vi "test-Diff-Drive-Accel-Limiter-Test1.vi"(8 "error in (no error)":errorcluster) -> (0 "error out":errorcluster, 3 "All tests passed":bool)   [LabVIEW 2019]
uses:
  <vilib>/Analysis/baseanly.llb/Real A x B.vi
  <vilib>/Rock Robotics/WPI/ThirdParty/JAS_Junk/TrajLib/MatBuilder_Create.vi
  <vilib>/Rock Robotics/WPI/ThirdParty/JAS_Junk/TrajLib/LinearSystem_New.vi
  <vilib>/Rock Robotics/WPI/ThirdParty/JAS_Junk/TrajLib/MatrixHelper_Zero.vi
  <vilib>/Rock Robotics/WPI/ThirdParty/JAS_Junk/TrajLib/Discretization_DiscretizeAB.vi
  <vilib>/Rock Robotics/WPI/ThirdParty/JAS_Junk/TrajLib/MatrixHelper_CoerceSize.vi
  <vilib>/Rock Robotics/WPI/ThirdParty/JAS_Junk/TrajLib/Matrix_Exp.vi
  <vilib>/Rock Robotics/WPI/ThirdParty/JAS_Junk/TrajLib/Matrix_AssignBlock.vi
  <vilib>/Rock Robotics/WPI/ThirdParty/JAS_Junk/TrajLib/Matrix_ExtractFrom.vi
  <vilib>/Analysis/7linalg.llb/Matrix Exp.vi
  <vilib>/Analysis/7linalg.llb/Real Matrix Exp.vi
  <vilib>/Analysis/Matrix/Numeric/Add/Add - RM,RM.vi
  <vilib>/Analysis/Matrix/Numeric/Multiply/Multiply.vi
  <vilib>/Analysis/Matrix/Numeric/Multiply/Multiply - RM,R.vi
  <vilib>/Rock Robotics/WPI/ThirdParty/JAS_Junk/TrajLib/Trajectory_Library.lvlib
  <vilib>/Analysis/NI_AALBase.lvlib
  <vilib>/Analysis/Matrix/NI_Matrix.lvlib
panel:
  out "max value 6":dbl
  out "max value 5":dbl
  out "max value 4":dbl
  out "max value 3":dbl
  out "max value 2":dbl
  out "max value":dbl
  out "Test 1":bool
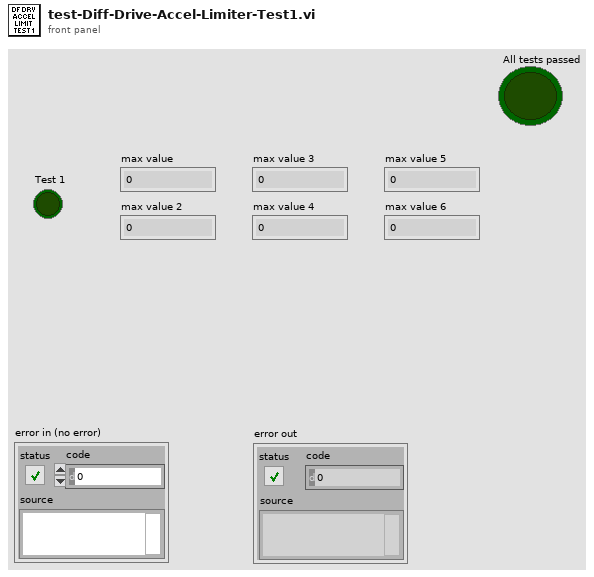
[diagram p1: front panel]
types:
  T1 = typedef "NI_Matrix.lvlib/RealMatrix.ctl" = dbl[][]
  T2 = typedef "Trajectory_Library.lvlib/LINEAR_SYSTEM.ctl" = cluster{"m_A":T1, "m_B":T1, "m_C":T1, "m_D":T1, "States":i32, "Inputs":i32, "Outputs":i32}
  T3 = typedef "Trajectory_Library.lvlib/DIFF_DRIVE_ACCEL_LIMIT.ctl" = cluster{"m_system":T2, "m_trackwidth":dbl, "m_maxLinearAccel":dbl, "m_maxAngularAccel":dbl}
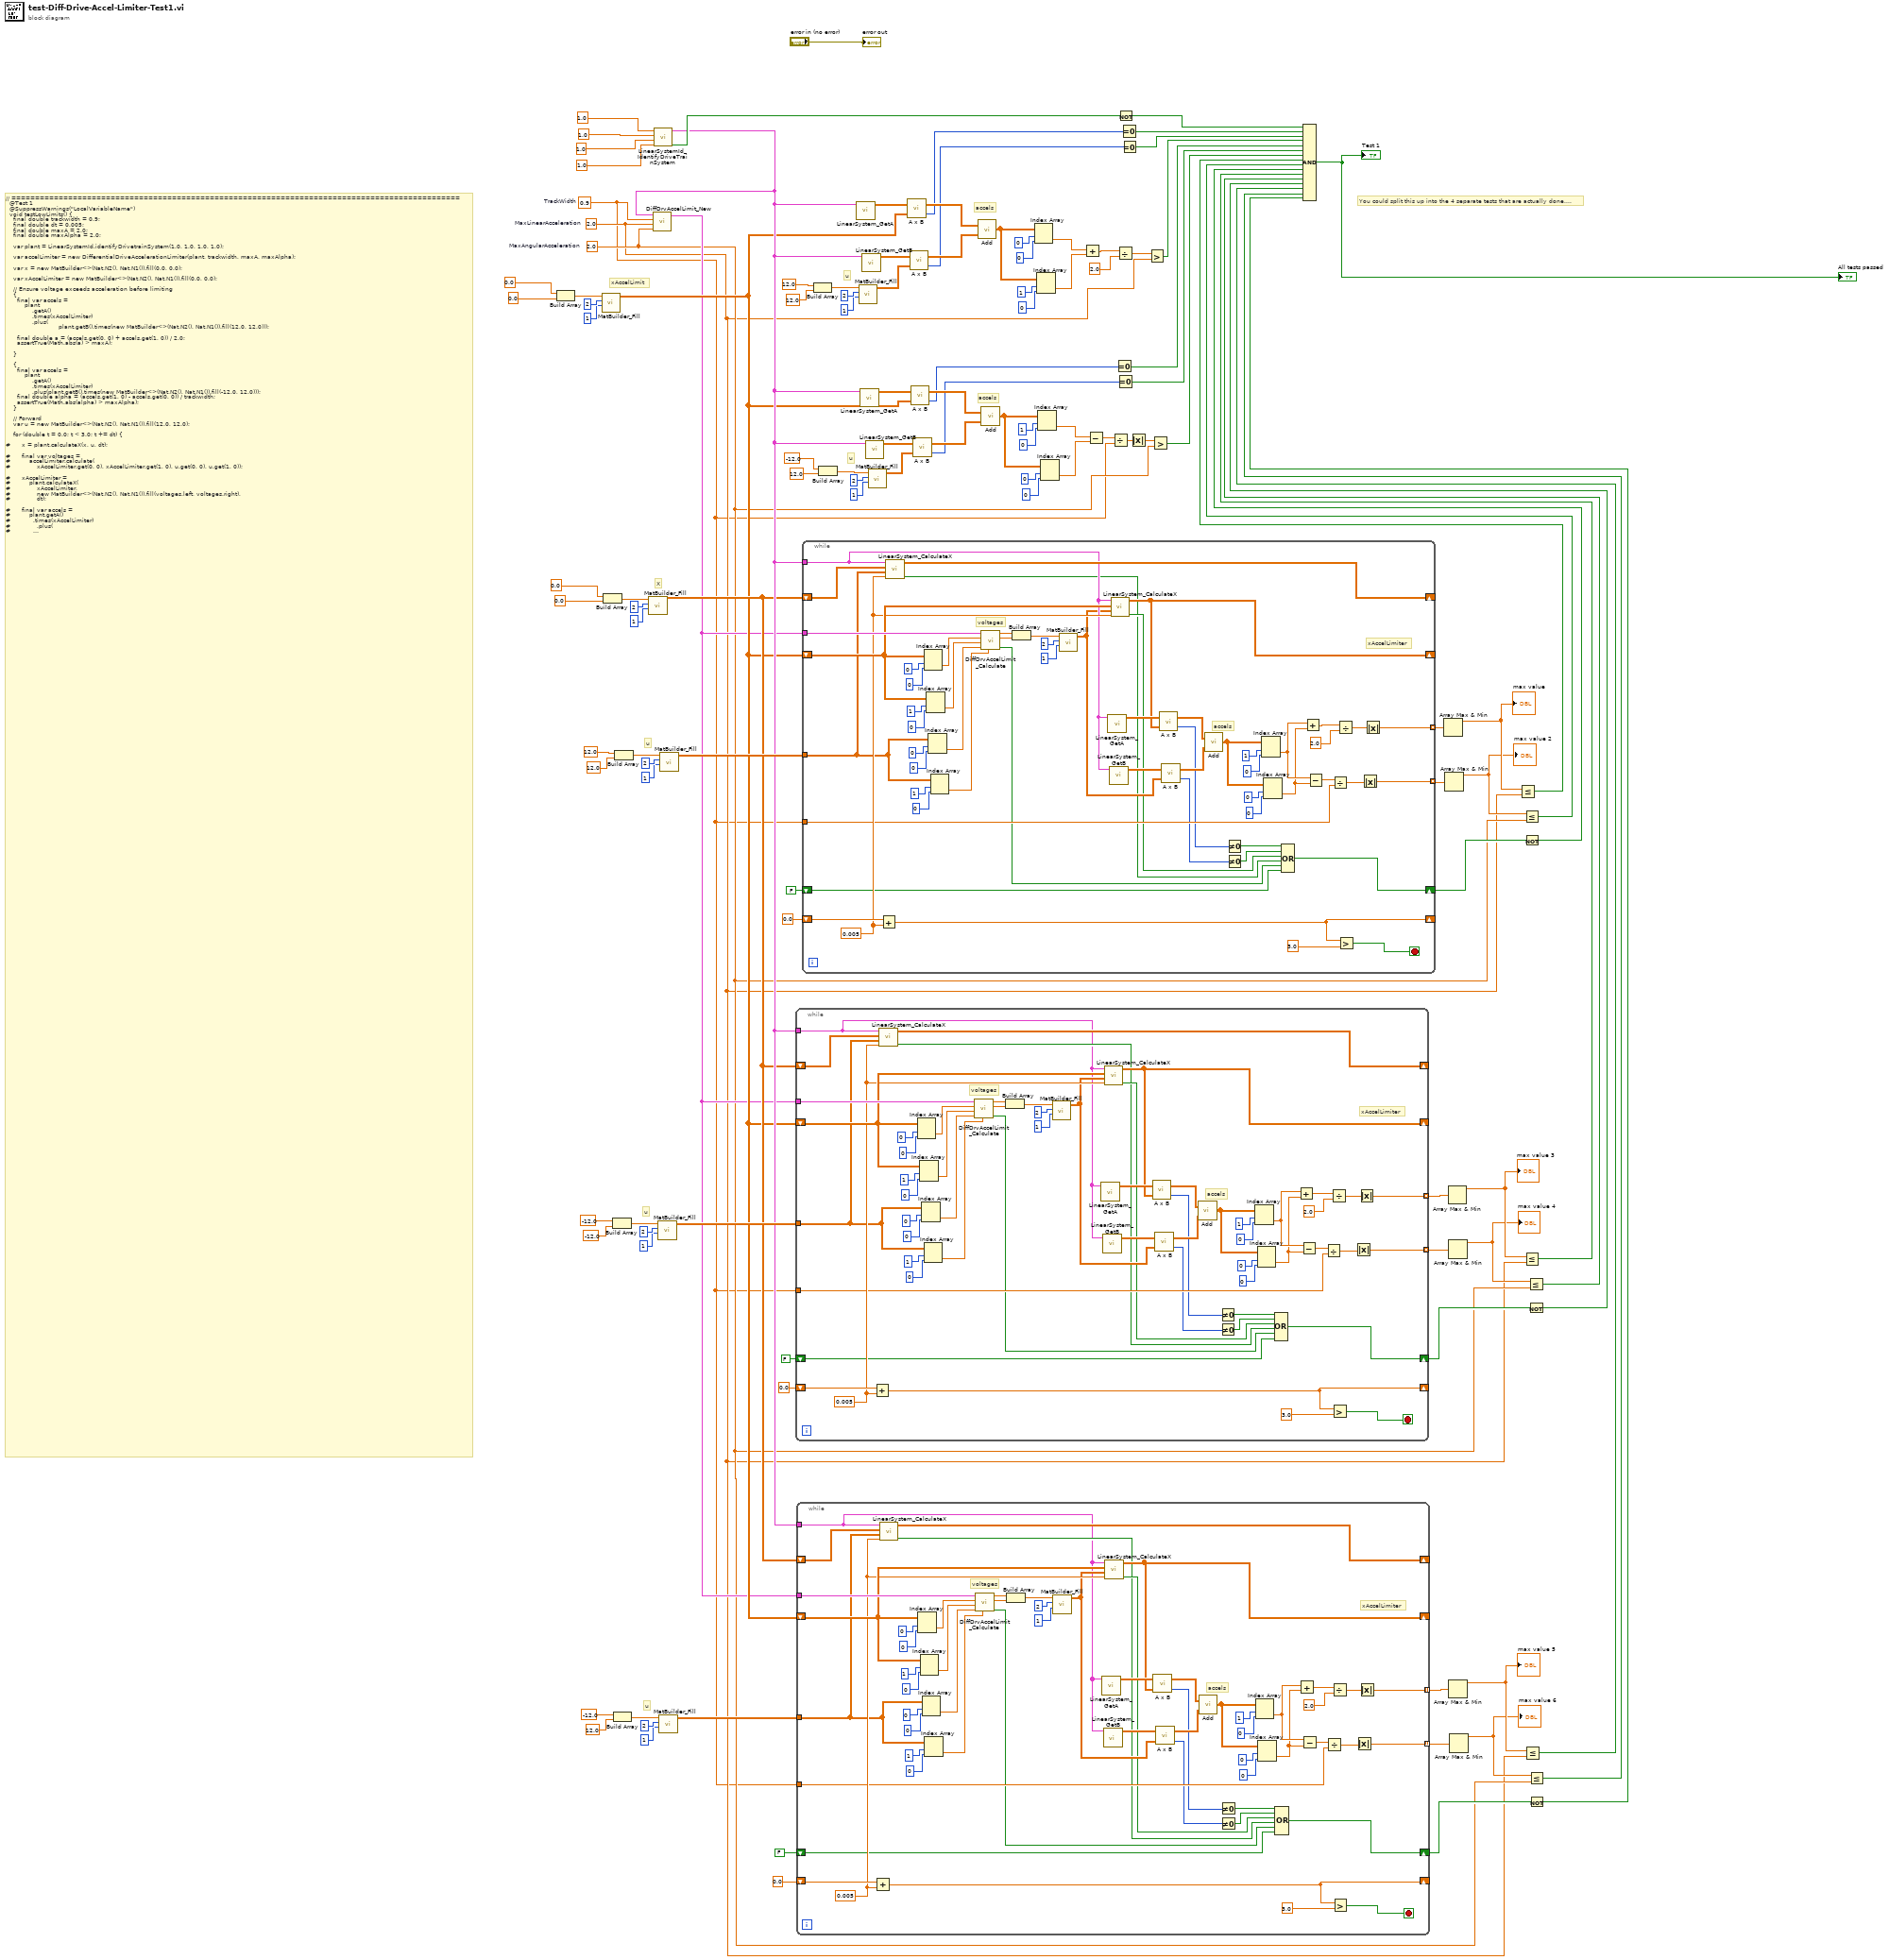
[diagram p0: block diagram]
diagram:
  w5 = 0.9  # TrackWidth
  w6 = 2.0  # MaxLinearAcceleration
  w7 = 2.0  # MaxAngularAcceleration
  # "You could split this up into the 4 separate tests that are actually done...."
  # "u"
  # "u"
  # "u"
  # "u"
  # "u"
  # "accels"
  # "accels"
  # "xAccelLimit"
  # "X"
  # "// ===============================================================================================\n  @Test 1\n  @SuppressWarnings(\"LocalVariableName\")\n  void testLowLimits() {\n    final double trackwidth = 0.9;\n    final double dt = 0.005;\n    final double maxA = 2.0;\n    final double maxAlpha = 2.0;\n\n    var plant = LinearSystemId.identifyDrivetrainSystem(1.0, 1.0, 1.0, 1.0);\n\n    var accelLimiter = new DifferentialDriveAccelerationLimiter(plant, trackwidth, maxA, maxAlpha);\n\n    var x = new MatBuilder<>(Nat.N2(), Nat.N1()).fill(0.0, 0.0);\n\n    var xAccelLimiter = new MatBuilder<>(Nat.N2(), Nat.N1()).fill(0.0, 0.0);\n\n    // Ensure voltage exceeds acceleration before limiting\n    {\n      final var accels =\n          plant\n              .getA()\n              .times(xAccelLimiter)\n              .plus(\n                            plant.getB().times(new MatBuilder<>(Nat.N2(), Nat.N1()).fill(12.0, 12.0)));\n\n      final double a = (accels.get(0, 0) + accels.get(1, 0)) / 2.0;\n      assertTrue(Math.abs(a) > maxA);\n\n    }\n\n    {\n      final var accels =\n          plant\n              .getA()\n              .times(xAccelLimiter)\n              .plus(plant.getB().times(new MatBuilder<>(Nat.N2(), Nat.N1()).fill(-12.0, 12.0)));\n      final double alpha = (accels.get(1, 0) - accels.get(0, 0)) / trackwidth;\n      assertTrue(Math.abs(alpha) > maxAlpha);\n    }\n\n    // Forward\n    var u = new MatBuilder<>(Nat.N2(), Nat.N1()).fill(12.0, 12.0);\n\n    for (double t = 0.0; t < 3.0; t += dt) {\n\n#      x = plant.calculateX(x, u, dt);\n\n#      final var voltages =\n#          accelLimiter.calculate(\n#              xAccelLimiter.get(0, 0), xAccelLimiter.get(1, 0), u.get(0, 0), u.get(1, 0));\n\n#      xAccelLimiter =\n#          plant.calculateX(\n#              xAccelLimiter,\n#              new MatBuilder<>(Nat.N2(), Nat.N1()).fill(voltages.left, voltages.right),\n#              dt);\n\n#      final var accels =\n#          plant.getA()\n#            .times(xAccelLimiter)\n#              .plus(\n#                  plant.getB()\n#                      .times(\n#                          new MatBuilder<>(Nat.N2(), Nat.N1())\n#                              .fill(voltages.left, voltages.right)));\n\n#      final double a = (accels.get(0, 0) + accels.get(1, 0)) / 2.0;\n\n#      final double alpha = (accels.get(1, 0) - accels.get(0, 0)) / trackwidth;\n\n#      assertTrue(Math.abs(a) <= maxA);\n#      assertTrue(Math.abs(alpha) <= maxAlpha);\n\n#    }\n\n    // Backward\n    u = new MatBuilder<>(Nat.N2(), Nat.N1()).fill(-12.0, -12.0);\n\n    for (double t = 0.0; t < 3.0; t += dt) {\n      x = plant.calculateX(x, u, dt);\n      final var voltages =\n          accelLimiter.calculate(\n              xAccelLimiter.get(0, 0), xAccelLimiter.get(1, 0), u.get(0, 0), u.get(1, 0));\n      xAccelLimiter =\n          plant.calculateX(\n              xAccelLimiter,\n              new MatBuilder<>(Nat.N2(), Nat.N1()).fill(voltages.left, voltages.right),\n              dt);\n\n      final var accels =\n          plant\n              .getA()\n              .times(xAccelLimiter)\n              .plus(\n                  plant\n                      .getB()\n                      .times(\n                          new MatBuilder<>(Nat.N2(), Nat.N1())\n                              .fill(voltages.left, voltages.right)));\n\n      final double a = (accels.get(0, 0) + accels.get(1, 0)) / 2.0;\n\n      final double alpha = (accels.get(1, 0) - accels.get(0, 0)) / trackwidth;\n\n      assertTrue(Math.abs(a) <= maxA);\n      assertTrue(Math.abs(alpha) <= maxAlpha);\n    }\n\n\n    // Rotate CCW\n    u = new MatBuilder<>(Nat.N2(), Nat.N1()).fill(-12.0, 12.0);\n    for (double t = 0.0; t < 3.0; t += dt) {\n      x = plant.calculateX(x, u, dt);\n      final var voltages =\n          accelLimiter.calculate(\n              xAccelLimiter.get(0, 0), xAccelLimiter.get(1, 0), u.get(0, 0), u.get(1, 0));\n      xAccelLimiter =\n          plant.calculateX(\n              xAccelLimiter,\n              new MatBuilder<>(Nat.N2(), Nat.N1()).fill(voltages.left, voltages.right),\n              dt);\n\n      final var accels =\n          plant\n              .getA()\n              .times(xAccelLimiter)\n              .plus(\n                  plant\n                      .getB()\n                      .times(\n                          new MatBuilder<>(Nat.N2(), Nat.N1())\n                              .fill(voltages.left, voltages.right)));\n      final double a = (accels.get(0, 0) + accels.get(1, 0)) / 2.0;\n      final double alpha = (accels.get(1, 0) - accels.get(0, 0)) / trackwidth;\n      assertTrue(Math.abs(a) <= maxA);\n      assertTrue(Math.abs(alpha) <= maxAlpha);\n    }\n  }"
  n1 = Build Array(0.0 ("element"), 0.0 ("element")) -> (w113:dbl[])
  n2 = call <vilib>:"MatBuilder_Fill.vi"("Columns"=1, "Rows"=2, "Value List"=w113) -> ("output matrix"=w9:T1)  [unwired: 8 in]
  n3 = Build Array(0.0 ("element"), 0.0 ("element")) -> (w118:dbl[])
  n4 = Build Array(-12.0 ("element"), -12.0 ("element")) -> (w38:dbl[])
  n5 = Build Array(-12.0 ("element"), 12.0 ("element")) -> (w22:dbl[])
  n6 = Build Array(12.0 ("element"), 12.0 ("element")) -> (w56:dbl[])
  n7 = call <vilib>:"MatBuilder_Fill.vi"("Columns"=1, "Rows"=2, "Value List"=w118) -> ("output matrix"=w10:T1)  [unwired: 8 in]
  n8 = call <vilib>:"LinearSystemId_IdentifyDriveTrainSystem.vi"("kAAngular"=1.0 ("rbMeters"), "kVAngular"=1.0 ("rMeters"), "kALinear"=1.0 ("MassKg"), "kVLinear"=1.0 ("JKgMetersSquared")) -> ("Size Coerced"=w93:bool, "Linearsystem"=w11:T2)  [unwired: 6 in]
  n9 = call <vilib>:"DiffDrvAccelLimit_New.vi"("MaxAngularAcceleration"=w7, "MaxLinearAcceleration"=w6, "TrackWidth"=w5, "LINEARSYSTEM"=w11) -> ("outDiffDriveAccelLimit"=w8:T3)  [unwired: 7 in]
  n10 = call <vilib>:"MatBuilder_Fill.vi"("Columns"=1, "Rows"=2, "Value List"=w38) -> ("output matrix"=w33:T1)  [unwired: 8 in]
  n11 = call <vilib>:"MatBuilder_Fill.vi"("Columns"=1, "Rows"=2, "Value List"=w22) -> ("output matrix"=w17:T1)  [unwired: 8 in]
  n12 = call <vilib>:"MatBuilder_Fill.vi"("Columns"=1, "Rows"=2, "Value List"=w56) -> ("output matrix"=w50:T1)  [unwired: 8 in]
  n13 = while {
    shift-right: [w178] -> _
    shift-left: 0.0 -> [w181]
    tunnel: w33 -> [w139]
    shift-right: [w171] -> _
    shift-left: w10 -> [w177]
    tunnel: w8 -> [w176]
    shift-right: [w146] -> _
    shift-left: w9 -> [w162]
    tunnel: w5 -> [w138]
    tunnel: [w135] -> w30 mode=indexing
    tunnel: [w134] -> w29 mode=indexing
    shift-right: [w125] -> w28
    shift-left: FALSE -> [w126]
    tunnel: w11 -> [w124]
    stop <- w180 stop-if-true
    w156 = 0.005
    # "voltages"
    # "xAccelLimiter"
    # "accels"
    n14 = Add(x=w181, y=w156) -> (x+y=w178:dbl)
    n15 = call <vilib>:"LinearSystem_CalculateX.vi"("dT_Seconds"=w156, "ClampedU"=w139, "X"=w177, "Linearsystem"=w124) -> ("Error"=w128:bool, "outX"=w171:T1)  [unwired: 6 in]
    n16 = Index Array(array=w162, index (row)=0, index (col)=0) -> (element=w170:dbl)
    n17 = Index Array(array=w162, index (row)=1, index (col)=0) -> (element=w169:dbl)
    n18 = Index Array(array=w139, index (row)=0, index (col)=0) -> (element=w164:dbl)
    n19 = Index Array(array=w139, index (row)=1, index (col)=0) -> (element=w163:dbl)
    n20 = call <vilib>:"DiffDrvAccelLimit_Calculate.vi"("RightVoltage"=w163, "LeftVoltage"=w164, "RightVelocity"=w169, "LeftVelocity"=w170, "inDiffDriveAccelLimit"=w176) -> ("Error"=w127:bool, "NewRightVoltage"=w157:dbl, "NewLeftVoltage"=w158:dbl)  [unwired: 4 in]
    n21 = Build Array(w158, w157) -> (w161:dbl[])
    n22 = call <vilib>:"MatBuilder_Fill.vi"("Columns"=1, "Rows"=2, "Value List"=w161) -> ("output matrix"=w145:T1)  [unwired: 8 in]
    n23 = call <vilib>:"LinearSystem_GetA.vi"("Linearsystem"=w124) -> ("A"=w155:T1)  [unwired: 10 in]
    n24 = call <vilib>:"LinearSystem_GetB.vi"("Linearsystem"=w124) -> ("B"=w154:T1)  [unwired: 10 in]
    n25 = call <vilib>:"LinearSystem_CalculateX.vi"("dT_Seconds"=w156, "ClampedU"=w145, "X"=w162, "Linearsystem"=w124) -> ("Error"=w129:bool, "outX"=w146:T1)  [unwired: 6 in]
    n26 = call-poly <vilib>:"A x B.vi"("B"=w146, "A"=w155) -> ("error"=w132:i32, "A x B"=w153:T1)
    n27 = call-poly <vilib>:"A x B.vi"("B"=w145, "A"=w154) -> ("error"=w131:i32, "A x B"=w152:T1)
    n28 = call-poly <vilib>:"Add.vi"("Real Matrix B"=w152, "Real Matrix A"=w153) -> ("A + B"=w147:T1)
    n29 = Not Equal To 0?(x=w132) -> (x != 0?=w133:bool)
    n30 = Not Equal To 0?(x=w131) -> (x != 0?=w130:bool)
    n31 = Index Array(array=w147, index (row)=1, index (col)=0) -> (element=w141:dbl)
    n32 = Index Array(array=w147, index (row)=0, index (col)=0) -> (element=w140:dbl)
    n33 = Compound Arithmetic op=OR(w133, w130, w129, w128, w127, w126) -> (w125:bool)
    n34 = Add(x=w141, y=w140) -> (x+y=w144:dbl)
    n35 = Subtract(x=w141, y=w140) -> (x-y=w142:dbl)
    n36 = Divide(x=w142, y=w138) -> (x/y=w136:dbl)
    n37 = Divide(x=w144, y=2.0) -> (x/y=w137:dbl)
    n38 = Greater?(x=w178, y=3.0) -> (0:w180:bool)
    n39 = Absolute Value(x=w136) -> (abs(x)=w134:dbl)
    n40 = Absolute Value(x=w137) -> (abs(x)=w135:dbl)
  }
  n41 = while {
    shift-right: [w236] -> _
    shift-left: 0.0 -> [w239]
    tunnel: w17 -> [w197]
    shift-right: [w229] -> _
    shift-left: w10 -> [w235]
    tunnel: w8 -> [w234]
    shift-right: [w204] -> _
    shift-left: w9 -> [w220]
    tunnel: w5 -> [w196]
    tunnel: [w193] -> w14 mode=indexing
    tunnel: [w192] -> w13 mode=indexing
    shift-right: [w183] -> w12
    shift-left: FALSE -> [w184]
    tunnel: w11 -> [w182]
    stop <- w238 stop-if-true
    w214 = 0.005
    # "voltages"
    # "xAccelLimiter"
    # "accels"
    n42 = Add(x=w239, y=w214) -> (x+y=w236:dbl)
    n43 = call <vilib>:"LinearSystem_CalculateX.vi"("dT_Seconds"=w214, "ClampedU"=w197, "X"=w235, "Linearsystem"=w182) -> ("Error"=w186:bool, "outX"=w229:T1)  [unwired: 6 in]
    n44 = Index Array(array=w220, index (row)=0, index (col)=0) -> (element=w228:dbl)
    n45 = Index Array(array=w220, index (row)=1, index (col)=0) -> (element=w227:dbl)
    n46 = Index Array(array=w197, index (row)=0, index (col)=0) -> (element=w222:dbl)
    n47 = Index Array(array=w197, index (row)=1, index (col)=0) -> (element=w221:dbl)
    n48 = call <vilib>:"DiffDrvAccelLimit_Calculate.vi"("RightVoltage"=w221, "LeftVoltage"=w222, "RightVelocity"=w227, "LeftVelocity"=w228, "inDiffDriveAccelLimit"=w234) -> ("Error"=w185:bool, "NewRightVoltage"=w215:dbl, "NewLeftVoltage"=w216:dbl)  [unwired: 4 in]
    n49 = Build Array(w216, w215) -> (w219:dbl[])
    n50 = call <vilib>:"MatBuilder_Fill.vi"("Columns"=1, "Rows"=2, "Value List"=w219) -> ("output matrix"=w203:T1)  [unwired: 8 in]
    n51 = call <vilib>:"LinearSystem_GetA.vi"("Linearsystem"=w182) -> ("A"=w213:T1)  [unwired: 10 in]
    n52 = call <vilib>:"LinearSystem_GetB.vi"("Linearsystem"=w182) -> ("B"=w212:T1)  [unwired: 10 in]
    n53 = call <vilib>:"LinearSystem_CalculateX.vi"("dT_Seconds"=w214, "ClampedU"=w203, "X"=w220, "Linearsystem"=w182) -> ("Error"=w187:bool, "outX"=w204:T1)  [unwired: 6 in]
    n54 = call-poly <vilib>:"A x B.vi"("B"=w204, "A"=w213) -> ("error"=w190:i32, "A x B"=w211:T1)
    n55 = call-poly <vilib>:"A x B.vi"("B"=w203, "A"=w212) -> ("error"=w189:i32, "A x B"=w210:T1)
    n56 = call-poly <vilib>:"Add.vi"("Real Matrix B"=w210, "Real Matrix A"=w211) -> ("A + B"=w205:T1)
    n57 = Not Equal To 0?(x=w190) -> (x != 0?=w191:bool)
    n58 = Not Equal To 0?(x=w189) -> (x != 0?=w188:bool)
    n59 = Index Array(array=w205, index (row)=1, index (col)=0) -> (element=w199:dbl)
    n60 = Index Array(array=w205, index (row)=0, index (col)=0) -> (element=w198:dbl)
    n61 = Compound Arithmetic op=OR(w191, w188, w187, w186, w185, w184) -> (w183:bool)
    n62 = Add(x=w199, y=w198) -> (x+y=w202:dbl)
    n63 = Subtract(x=w199, y=w198) -> (x-y=w200:dbl)
    n64 = Divide(x=w200, y=w196) -> (x/y=w194:dbl)
    n65 = Divide(x=w202, y=2.0) -> (x/y=w195:dbl)
    n66 = Greater?(x=w236, y=3.0) -> (0:w238:bool)
    n67 = Absolute Value(x=w194) -> (abs(x)=w192:dbl)
    n68 = Absolute Value(x=w195) -> (abs(x)=w193:dbl)
  }
  n69 = while {
    shift-right: [w294] -> _
    shift-left: 0.0 -> [w297]
    tunnel: w11 -> [w262]
    tunnel: w50 -> [w254]
    shift-right: [w287] -> _
    shift-left: w10 -> [w293]
    tunnel: w8 -> [w292]
    shift-right: [w261] -> _
    shift-left: w9 -> [w278]
    tunnel: w5 -> [w253]
    tunnel: [w250] -> w49 mode=indexing
    tunnel: [w249] -> w48 mode=indexing
    shift-right: [w240] -> w44
    shift-left: FALSE -> [w241]
    stop <- w296 stop-if-true
    w272 = 0.005
    # "voltages"
    # "xAccelLimiter"
    # "accels"
    n70 = Add(x=w297, y=w272) -> (x+y=w294:dbl)
    n71 = call <vilib>:"LinearSystem_CalculateX.vi"("dT_Seconds"=w272, "ClampedU"=w254, "X"=w293, "Linearsystem"=w262) -> ("Error"=w243:bool, "outX"=w287:T1)  [unwired: 6 in]
    n72 = Index Array(array=w278, index (row)=0, index (col)=0) -> (element=w286:dbl)
    n73 = Index Array(array=w278, index (row)=1, index (col)=0) -> (element=w285:dbl)
    n74 = Index Array(array=w254, index (row)=0, index (col)=0) -> (element=w280:dbl)
    n75 = Index Array(array=w254, index (row)=1, index (col)=0) -> (element=w279:dbl)
    n76 = call <vilib>:"DiffDrvAccelLimit_Calculate.vi"("RightVoltage"=w279, "LeftVoltage"=w280, "RightVelocity"=w285, "LeftVelocity"=w286, "inDiffDriveAccelLimit"=w292) -> ("Error"=w242:bool, "NewRightVoltage"=w273:dbl, "NewLeftVoltage"=w274:dbl)  [unwired: 4 in]
    n77 = Build Array(w274, w273) -> (w277:dbl[])
    n78 = call <vilib>:"MatBuilder_Fill.vi"("Columns"=1, "Rows"=2, "Value List"=w277) -> ("output matrix"=w260:T1)  [unwired: 8 in]
    n79 = call <vilib>:"LinearSystem_GetA.vi"("Linearsystem"=w262) -> ("A"=w271:T1)  [unwired: 10 in]
    n80 = call <vilib>:"LinearSystem_GetB.vi"("Linearsystem"=w262) -> ("B"=w270:T1)  [unwired: 10 in]
    n81 = call <vilib>:"LinearSystem_CalculateX.vi"("dT_Seconds"=w272, "ClampedU"=w260, "X"=w278, "Linearsystem"=w262) -> ("Error"=w244:bool, "outX"=w261:T1)  [unwired: 6 in]
    n82 = call-poly <vilib>:"A x B.vi"("B"=w261, "A"=w271) -> ("error"=w247:i32, "A x B"=w269:T1)
    n83 = call-poly <vilib>:"A x B.vi"("B"=w260, "A"=w270) -> ("error"=w246:i32, "A x B"=w268:T1)
    n84 = call-poly <vilib>:"Add.vi"("Real Matrix B"=w268, "Real Matrix A"=w269) -> ("A + B"=w263:T1)
    n85 = Not Equal To 0?(x=w247) -> (x != 0?=w248:bool)
    n86 = Not Equal To 0?(x=w246) -> (x != 0?=w245:bool)
    n87 = Index Array(array=w263, index (row)=1, index (col)=0) -> (element=w256:dbl)
    n88 = Index Array(array=w263, index (row)=0, index (col)=0) -> (element=w255:dbl)
    n89 = Compound Arithmetic op=OR(w248, w245, w244, w243, w242, w241) -> (w240:bool)
    n90 = Add(x=w256, y=w255) -> (x+y=w259:dbl)
    n91 = Subtract(x=w256, y=w255) -> (x-y=w257:dbl)
    n92 = Divide(x=w257, y=w253) -> (x/y=w251:dbl)
    n93 = Divide(x=w259, y=2.0) -> (x/y=w252:dbl)
    n94 = Greater?(x=w294, y=3.0) -> (0:w296:bool)
    n95 = Absolute Value(x=w251) -> (abs(x)=w249:dbl)
    n96 = Absolute Value(x=w252) -> (abs(x)=w250:dbl)
  }
  n97 = Build Array(12.0 ("element"), 12.0 ("element")) -> (w106:dbl[])
  n98 = Build Array(-12.0 ("element"), 12.0 ("element")) -> (w69:dbl[])
  n99 = call <vilib>:"LinearSystem_GetA.vi"("Linearsystem"=w11) -> ("A"=w108:T1)  [unwired: 10 in]
  n100 = call <vilib>:"MatBuilder_Fill.vi"("Columns"=1, "Rows"=2, "Value List"=w106) -> ("output matrix"=w101:T1)  [unwired: 8 in]
  n101 = call <vilib>:"LinearSystem_GetA.vi"("Linearsystem"=w11) -> ("A"=w81:T1)  [unwired: 10 in]
  n102 = call <vilib>:"LinearSystem_GetB.vi"("Linearsystem"=w11) -> ("B"=w107:T1)  [unwired: 10 in]
  n103 = call <vilib>:"LinearSystem_GetB.vi"("Linearsystem"=w11) -> ("B"=w80:T1)  [unwired: 10 in]
  n104 = call <vilib>:"MatBuilder_Fill.vi"("Columns"=1, "Rows"=2, "Value List"=w69) -> ("output matrix"=w64:T1)  [unwired: 8 in]
  n105 = call-poly <vilib>:"A x B.vi"("B"=w9, "A"=w108) -> ("error"=w91:i32, "A x B"=w100:T1)
  n106 = call-poly <vilib>:"A x B.vi"("B"=w101, "A"=w107) -> ("error"=w90:i32, "A x B"=w99:T1)
  n107 = call-poly <vilib>:"A x B.vi"("B"=w9, "A"=w81) -> ("error"=w63:i32, "A x B"=w79:T1)
  n108 = call-poly <vilib>:"A x B.vi"("B"=w64, "A"=w80) -> ("error"=w62:i32, "A x B"=w78:T1)
  n109 = call-poly <vilib>:"Add.vi"("Real Matrix B"=w99, "Real Matrix A"=w100) -> ("A + B"=w94:T1)
  n110 = call-poly <vilib>:"Add.vi"("Real Matrix B"=w78, "Real Matrix A"=w79) -> ("A + B"=w73:T1)
  n111 = Index Array(array=w94, index (row)=0, index (col)=0) -> (element=w87:dbl)
  n112 = Index Array(array=w94, index (row)=1, index (col)=0) -> (element=w86:dbl)
  n113 = Index Array(array=w73, index (row)=1, index (col)=0) -> (element=w72:dbl)
  n114 = Index Array(array=w73, index (row)=0, index (col)=0) -> (element=w71:dbl)
  n115 = Add(x=w87, y=w86) -> (x+y=w85:dbl)
  n116 = Subtract(x=w72, y=w71) -> (x-y=w70:dbl)
  n117 = Divide(x=w70, y=w5) -> (x/y=w61:dbl)
  n118 = Equal To 0?(x=w63) -> (x = 0?=w59:bool)
  n119 = Divide(x=w85, y=2.0) -> (x/y=w83:dbl)
  n120 = Equal To 0?(x=w62) -> (x = 0?=w58:bool)
  n121 = Not(x=w93) -> (.not. x?=w92:bool)
  n122 = Equal To 0?(x=w91) -> (x = 0?=w89:bool)
  n123 = Equal To 0?(x=w90) -> (x = 0?=w88:bool)
  n124 = Absolute Value(x=w61) -> (abs(x)=w60:dbl)
  n125 = Greater?(x=w83, y=w6) -> (0:w82:bool)
  n126 = Greater?(x=w60, y=w7) -> (0:w57:bool)
  n127 = Array Max & Min(array=w49) -> (max value=w47:dbl)  [unwired: 3 out]
  "max value" <- w47
  n128 = Array Max & Min(array=w48) -> (max value=w46:dbl)  [unwired: 3 out]
  "max value 2" <- w46
  n129 = Array Max & Min(array=w30) -> (max value=w32:dbl)  [unwired: 3 out]
  "max value 3" <- w32
  n130 = Array Max & Min(array=w29) -> (max value=w31:dbl)  [unwired: 3 out]
  "max value 4" <- w31
  n131 = Array Max & Min(array=w14) -> (max value=w16:dbl)  [unwired: 3 out]
  "max value 5" <- w16
  n132 = Array Max & Min(array=w13) -> (max value=w15:dbl)  [unwired: 3 out]
  "max value 6" <- w15
  n133 = Less Or Equal?(x=w47, y=w6) -> (x <= y?=w43:bool)
  n134 = Less Or Equal?(x=w46, y=w7) -> (x <= y?=w42:bool)
  n135 = Not(x=w44) -> (.not. x?=w41:bool)
  n136 = Less Or Equal?(x=w32, y=w6) -> (x <= y?=w27:bool)
  n137 = Less Or Equal?(x=w16, y=w6) -> (x <= y?=w4:bool)
  n138 = Less Or Equal?(x=w31, y=w7) -> (x <= y?=w26:bool)
  n139 = Not(x=w28) -> (.not. x?=w25:bool)
  n140 = Less Or Equal?(x=w15, y=w7) -> (x <= y?=w3:bool)
  n141 = Not(x=w12) -> (.not. x?=w2:bool)
  n142 = Compound Arithmetic op=AND(w92, w89, w88, w82, w59, w58, w57, w43, w42, w41, w27, w26, w25, w4, w3, w2) -> (→"All tests passed" →"Test 1":bool)
  "error out" <- "error in (no error)"
